vi "Set Keyprotect.vi"(7 "Keyprotect (On/Off)":bool, 8 "error in (no error)":errorcluster, 10 "Address (0)":i32, 11 "VISA resource name":refnum<visa-resource-name>) -> (0 "error out":errorcluster, 3 "VISA resource name out":refnum<visa-resource-name>)   [LabVIEW 2016, in "Environment Chamber.lvlib" / "Climatic Chamber.lvlib"]
doc: "<b>Key protection setting</B>\n\nEnables or Disables setting change protection and operation protection at the same time."
uses:
  Climatic Chamber.lvlib
panel:
  out "NACK":bool
  out "Error":bool
  out "ACK":bool
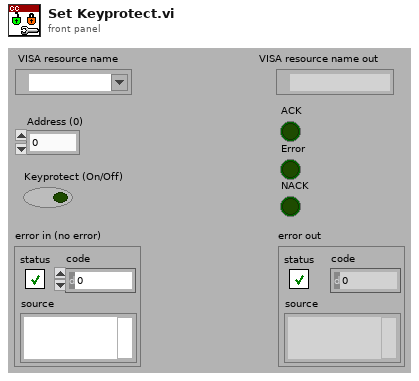
[diagram p1: front panel]
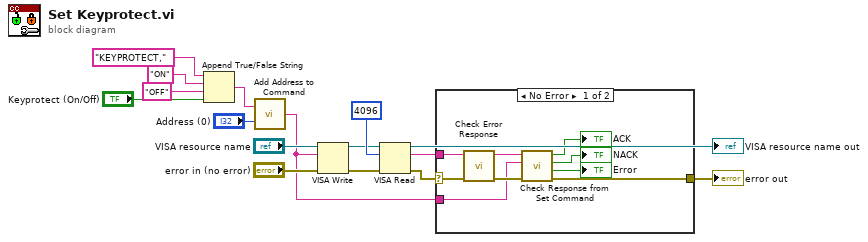
[diagram p0: block diagram]
diagram:
  n1 = Append True/False String(1:"Keyprotect (On/Off)", 2:"OFF", 3:"ON", 4:"KEYPROTECT," ("string (\"\")")) -> (0:w1:string)
  n2 = call "Add Address to Command.vi"("Address (0)"="Address (0)", "Command"=w1) -> ("Command OUT"=w6:string)
  n3 = VISA Write(VISA resource name="VISA resource name", write buffer=w6, error in (no error)="error in (no error)") -> (VISA resource name out=w13:refnum<visa-resource-name>, error out=w12:errorcluster)  [unwired: 1 out]
  n4 = VISA Read(VISA resource name=w13, byte count=u32 4096, error in (no error)=w12) -> (VISA resource name out=→"VISA resource name out":refnum<visa-resource-name>, read buffer=w8:string, error out=w9:errorcluster)  [unwired: 1 out]
  n5 = case shown="No Error" w9 {
    selector: w9 -> [w24 w26]
    tunnel: w8 -> [w25 _]
    tunnel: [w20 w26] -> w7
    tunnel: w6 -> [w21 _]
    frame No Error {
      n6 = call "Check Error Response.vi"("error in (no error)"=w24, "read String"=w25) -> ("error out"=w23:errorcluster, "String out"=w22:string)  [unwired: 7 in, 1 out]
      n7 = call "Check Response from Set Command.vi"("error in (no error)"=w23, "Command"=w21, "Response"=w22) -> ("error out"=w20:errorcluster, "Error"=→"Error":bool, "NACK"=→"NACK":bool, "ACK"=→"ACK":bool)  [unwired: 5 in]
    }
    frame Error {
    }
  }
  "error out" <- w7
